vi "Thermocouple_DAQ_read.vi"() -> ()   [LabVIEW 2021]
uses:
  <vilib>/DAQmx/read.llb/DAQmx Read (Analog 1D DBL NChan 1Samp).vi
  <vilib>/Utility/file.llb/Write Delimited Spreadsheet (string).vi
  <vilib>/DAQmx/miscellaneous.llb/DAQmx Fill In Error Info.vi
panel:
  out "latest save":string
  out "Runtime [s]":dbl
  out "iter":i32
  in  "cycle time [s]":u32=2000
  in  "file path (dialog if empty) 2":path=path "C:/Users/wendell/Documents/GitHub/CFD_test/CFD_data/test.csv"
  out "file path (dialog if empty)":path=path "C:/Users/wendell/Documents/GitHub/CFD_test/CFD_data.csv"
  out "data":dbl[](array[numeric]) format="%0.2f"
  in  "stop":bool
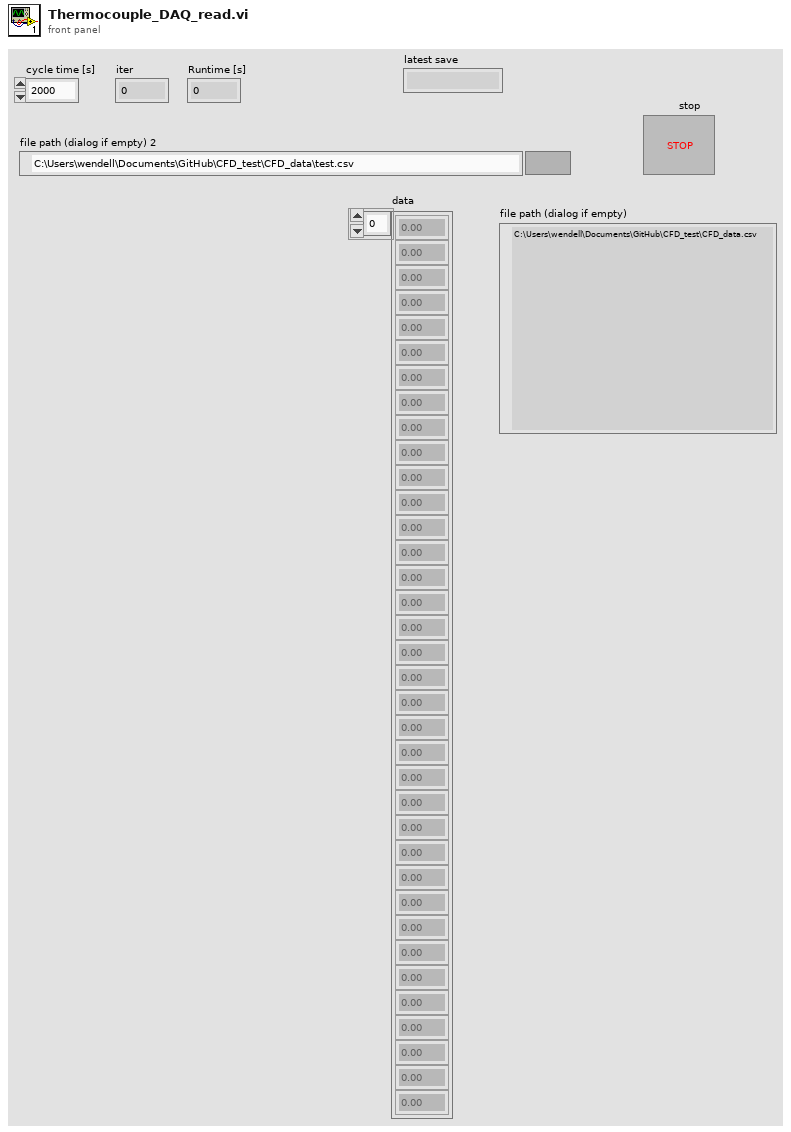
[diagram p1: front panel]
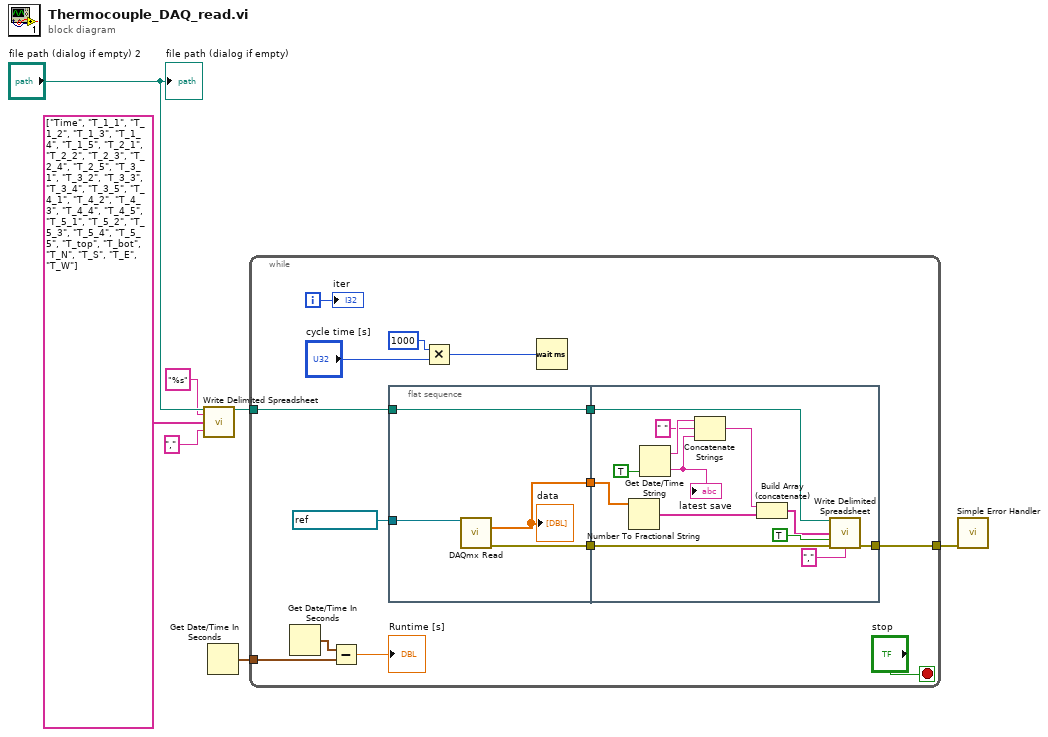
[diagram p0: block diagram]
diagram:
  n1 = call-poly <vilib>:"Write Delimited Spreadsheet.vi"("file path (dialog if empty)"="file path (dialog if empty) 2", "format (%s)"="%s" ("format (%.3f)"), "1D data"=string[] ["Time", "T_1_1", "T_1_2", "T_1_3", "T_1_4", "T_1_5", "T_2_1", "T_2_2", "T_2_3", "T_2_4", "T_2_5", "T_3_1", "T_3_2", "T_3_3", "T_3_4", "T_3_5", "T_4_1", "T_4_2", "T_4_3", "T_4_4", "T_4_5", "T_5_1", "T_5_2", "T_5_3", "T_5_4", "T_5_5", "T_top", "T_bot", "T_N", "T_S", "T_E", "T_W"], "delimiter (\\t)"="," ("delimiter (\\t)")) -> ("new file path (Not A Path if cancelled)"=w2:path)  [unwired: 10 in, 1 out]
  n2 = Get Date/Time In Seconds() -> (seconds since 1Jan1904=w1:timestamp)
  n3 = while {
    tunnel: [w19] -> w7
    tunnel: w2 -> [w15]
    tunnel: w1 -> [w9]
    i -> [w11]
    stop <- "stop" stop-if-true
    n4 = Get Date/Time In Seconds() -> (seconds since 1Jan1904=w10:timestamp)
    n5 = Subtract(x=w10, y=w9) -> (x-y=→"Runtime [s]":dbl)
    n6 = flat-sequence {
      tunnel: [w25] -> w21
      tunnel: [w24] -> w20
      tunnel: [w22] -> w17
      tunnel: refnum<k21> "CFD_Temp" ("task/channels in") -> [w23]
      tunnel: w15 -> [w22]
      tunnel: w21 -> [w33]
      tunnel: w20 -> [w38]
      tunnel: [w37] -> w19
      tunnel: w17 -> [w36]
      frame #0 {
        n7 = call-poly <vilib>:"DAQmx Read.vi"("task/channels in"=w23) -> ("data"=w25:dbl[], "error out"=w24:errorcluster)  [unwired: 12 in, 1 out]
        "data" <- w25
      }
      frame #1 {
        n8 = Number To Fractional String(number=w33) -> (F-format string=w32:string[])  [unwired: 3 in]
        n9 = Get Date/Time String(want seconds? (F)=TRUE) -> (date string=w29:string, time string=w27:string)  [unwired: 2 in]
        "latest save" <- w27
        n10 = Concatenate Strings(w29, " " ("string"), w27) -> (w28:string)
        n11 = Build Array (concatenate)(w28, w32) -> (w31:string[])
        n12 = call-poly <vilib>:"Write Delimited Spreadsheet.vi"("file path (dialog if empty)"=w36, "1D data"=w31, "append to file? (new file:F)"=TRUE, "error in (no error)"=w38, "delimiter (\\t)"="," ("delimiter (\\t)")) -> ("error out"=w37:errorcluster)  [unwired: 9 in, 1 out]
      }
    }
    n13 = Multiply(x=u32 1000, y="cycle time [s]") -> (x*y=w12:u32)
    n14 = Wait (ms)(milliseconds to wait=w12) -> ()  [unwired: 1 out]
    "iter" <- w11
  }
  n15 = call <vilib>:"Simple Error Handler.vi"("error in (no error)"=w7) -> ()  [unwired: 4 in, 5 out]
  "file path (dialog if empty)" <- "file path (dialog if empty) 2"
